vi "XIPIN_JTAG_to_AXI_Master_1_1.vi"   [LabVIEW 2017]
doc: "JTAG to AXI Master generates AXI transactions. The AXI transactions are generated by issuing write and read commands from JTAG.\n------------------------------------\n<b>Need License</b> : No\n<b>Interface</b> : AXI4"
uses:
  <vilib>/rvi/XilinxIP/XIPIN_XNode/niFpgaXIPIN.xnode
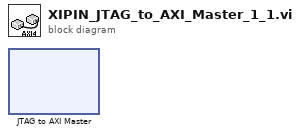
[diagram p0: block diagram]
diagram:
  n1 = xnode ("JTAG to AXI Master")() -> ()
